vi "MM_ConnectControlsToCP.vi"(8 "error in (no error)":errorcluster, 9 "Wiring Rules":T1(array[ring]), 10 "Controls":refnum<vi>[](array[refnum]), 11 "vi ref in":refnum<vi>) -> (0 "error out":errorcluster, 3 "vi ref out":refnum<vi>)   [LabVIEW 2012]
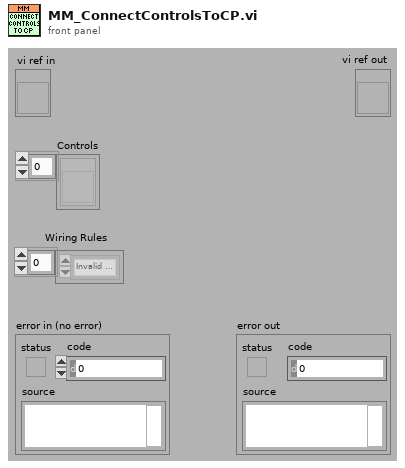
[diagram p1: front panel]
types:
  T1 = enum16{"Invalid Wire Rule", "Required", "Recommended", "Optional", "Dynamic Dispatch"}[]
  T2 = enum16{"Invalid Wire Rule", "Required", "Recommended", "Optional", "Dynamic Dispatch"}
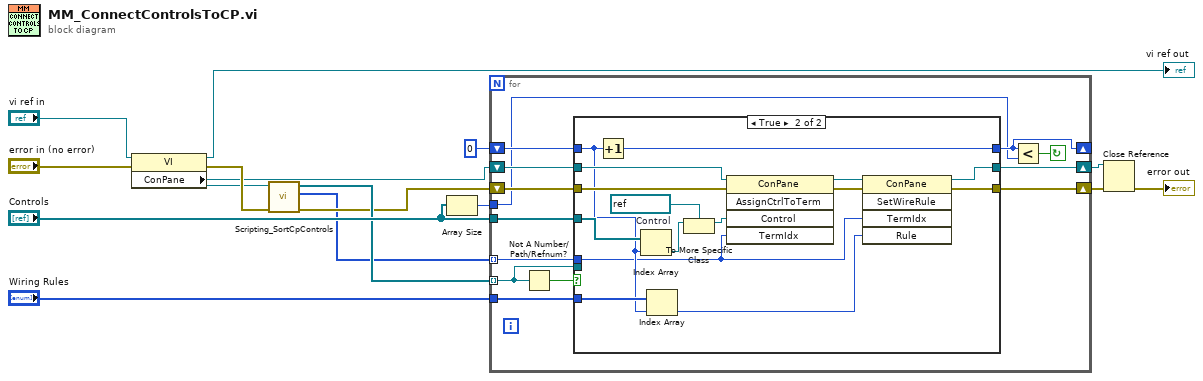
[diagram p0: block diagram]
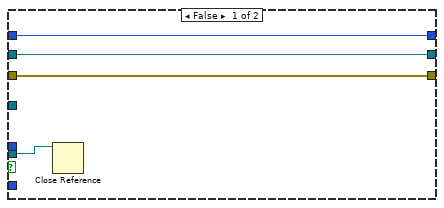
[diagram p2: hidden frame]
diagram:
  n1 = property class="VI"(reference="vi ref in", error in="error in (no error)") -> (reference out=→"vi ref out":refnum<vi>, error out=w5:errorcluster, "ConPane"=w4:refnum<vi>)
  n2 = call <resource>:"Scripting_SortCpControls.vi"("error in (no error)"=w5, "Connector Pane:Reference"=w4) -> ("error out"=w2:errorcluster, "TermIndex"=w1:i32[], "Controls[]"=w3:refnum<vi>[])  [unwired: 4 in, 3 out]
  n3 = Array Size(array="Controls") -> (size(s)=w14:i32)
  n4 = for {
    tunnel: w3 -> [w17] mode=indexing
    shift-right: [w27] -> w9
    shift-left: w4 -> [w28]
    shift-right: [w25] -> w8
    shift-left: w2 -> [w26]
    tunnel: "Controls" -> [w23]
    shift-right: [w20] -> _
    shift-left: 0 ("index") -> [w22]
    tunnel: w14 -> [w19]
    tunnel: "Wiring Rules" -> [w18]
    tunnel: w1 -> [w16] mode=indexing
    stop <- w21 continue-if-true
    n5 = Not A Number/Path/Refnum?(number/path/refnum=w17) -> (NaN/Path/Refnum?=w24:bool)
    n6 = case shown="True" w24 {
      tunnel: w28 -> [w32 w47]
      tunnel: [w32 w37] -> w27
      tunnel: w26 -> [w31 w46]
      tunnel: [w31 w38] -> w25
      tunnel: w23 -> [_ w45]
      tunnel: w22 -> [w30 w35]
      tunnel: [w30 w44] -> w20
      tunnel: w18 -> [_ w36]
      tunnel: w17 -> [w29 _]
      tunnel: w16 -> [_ w33]
      frame False {
        n7 = Close Reference(reference=w29) -> ()  [unwired: 1 in, 1 out]
      }
      frame True {
        w42 = refnum<vi> refnum  # Control
        n8 = Increment(x=w35) -> (x+1=w44:i32)
        n9 = Index Array(array=w45, index=w35) -> (element=w43:refnum<vi>)
        n10 = Index Array(array=w36, index=w35) -> (element=w34:T2)
        n11 = To More Specific Class(target class=w42, reference=w43) -> (specific class reference=w41:refnum<vi>)  [unwired: 1 in, 1 out]
        n12 = invoke class="ConPane" method="AssignCtrlToTerm"(reference=w47, error in=w46, "Control"=w41, "TermIdx"=w33) -> (reference out=w40:refnum<vi>, error out=w39:errorcluster)  [unwired: 1 in, 3 out]
        n13 = invoke class="ConPane" method="SetWireRule"(reference=w40, error in=w39, "TermIdx"=w33, "Rule"=w34) -> (reference out=w37:refnum<vi>, error out=w38:errorcluster)  [unwired: 1 in, 3 out]
      }
    }
    n14 = Less?(x=w20, y=w19) -> (x < y?=w21:bool)
  }
  n15 = Close Reference(reference=w9, error in (no error)=w8) -> (error out=→"error out":errorcluster)
